vi "Construct Read Transfer State SHV.vi"(8 "error in (no error)":errorcluster) -> (0 "error out":errorcluster, 2 "State":T1)   [LabVIEW 2015]
uses:
  Controls/Sample Transfer State Enumerator.ctl
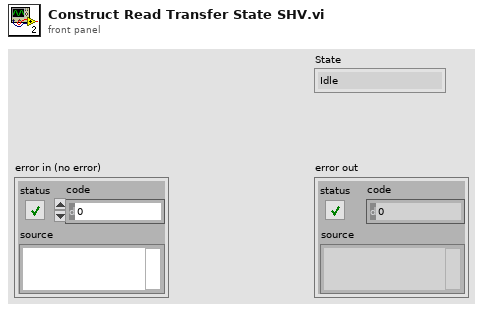
[diagram p1: front panel]
types:
  T1 = typedef "Sample Transfer State Enumerator.ctl" = enum16{"Idle", "Initialize", "Check Containers", "Check Temperatures", "Start Turbo", "Warm Up Containers", "Prepare for purging", "Purge Capillary", "Purge", "Open Containers", "Introduce Sample", "Measure Base Pressure", "Home Syringe", "Start Freezer", "Freeze Target", "Crystalize", "Stash", "Polish", "Stop Freezers", "Push Sample", "Complete", "Abort", "Error", "Undefined"}
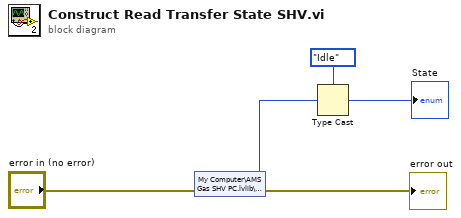
[diagram p0: block diagram]
diagram:
  n1 = shared-variable "My Computer\\AMS Gas SHV PC.lvlib\\Sample Transfer.lvlib\\State"(error in="error in (no error)") -> (w3:u16, error out=→"error out":errorcluster)
  n2 = Type Cast(type=Sample_Transfer_State_Enumerator."Idle" ("State"), x=w3) -> (*(type *) &x=→"State":T1)
